vi "RF_Synth_read.vi"(1 "Parameter":T1(ring), 2 "Address":string) -> (0 "Value":dbl)   [LabVIEW 2013]
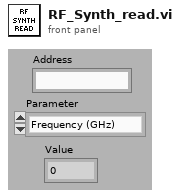
[diagram p1: front panel]
types:
  T1 = enum16{"Frequency (GHz)", "Power (dBm)", "Phase (deg)", "Output on?"}
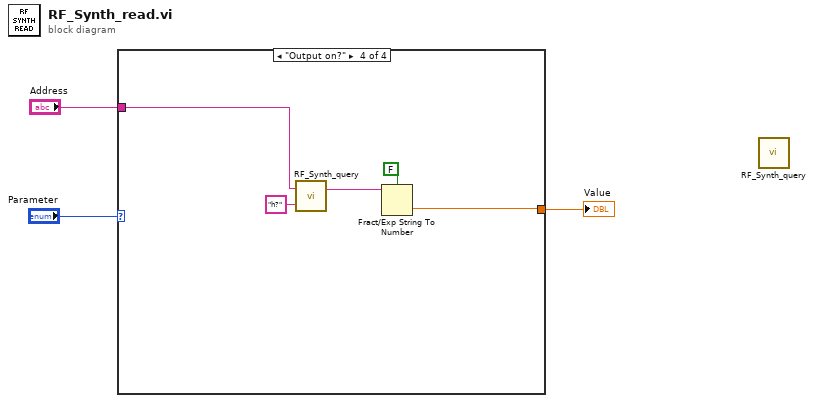
[diagram p0: block diagram]
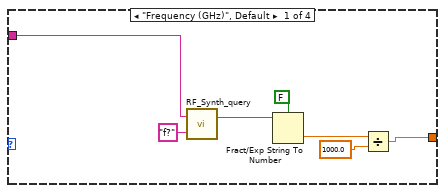
[diagram p2: hidden frame]
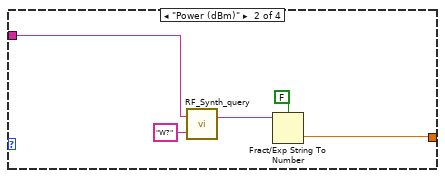
[diagram p3: hidden frame]
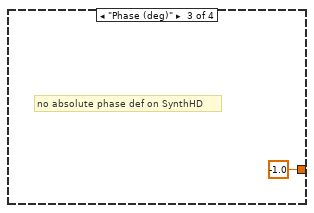
[diagram p4: hidden frame]
diagram:
  n1 = case shown="\"Output on?\"" "Parameter" {
    tunnel: [w5 w11 -1.0 w17] -> w2
    tunnel: "Address" -> [w10 w15 _ w21]
    frame "Frequency (GHz)", Default {
      n2 = call "RF_Synth_query.vi"("write buffer"="f?", "VISA resource name"=w10) -> ("read buffer"=w7:string)  [unwired: 1 out]
      n3 = Fract/Exp String To Number(use system decimal point (T)=FALSE, string=w7) -> (number=w6:dbl)  [unwired: 2 in, 1 out]
      n4 = Divide(x=w6, y=1000.0) -> (x/y=w5:dbl)
    }
    frame "Power (dBm)" {
      n5 = call "RF_Synth_query.vi"("write buffer"="W?", "VISA resource name"=w15) -> ("read buffer"=w12:string)  [unwired: 1 out]
      n6 = Fract/Exp String To Number(use system decimal point (T)=FALSE, string=w12) -> (number=w11:dbl)  [unwired: 2 in, 1 out]
    }
    frame "Phase (deg)" {
      # "no absolute phase def on SynthHD"
    }
    frame "Output on?" {
      n7 = call "RF_Synth_query.vi"("write buffer"="h?", "VISA resource name"=w21) -> ("read buffer"=w18:string)  [unwired: 1 out]
      n8 = Fract/Exp String To Number(use system decimal point (T)=FALSE, string=w18) -> (number=w17:dbl)  [unwired: 2 in, 1 out]
    }
  }
  "Value" <- w2
  n9 = call "RF_Synth_query.vi"() -> ()  [unwired: 2 in, 2 out]
